vi "Measure_Power_Good.vi"(8 "error in (no error)":errorcluster, 10 "Parameters":string, 11 "reference in":refnum<class "Test_Flux_Capacitor.lvclass">) -> (0 "error out":errorcluster, 2 "Result":dbl, 3 "reference out":refnum<class "Test_Flux_Capacitor.lvclass">)   [LabVIEW 2022 SP3, in "Test_Flux_Capacitor.lvlib" / "Test_Flux_Capacitor.lvclass"]
uses:
  Test_Flux_Capacitor.lvclass
  ParameterTypes/PowerGood.ctl
  ParameterTypes/DMM_DCV.vi
  <vilib>/Analysis/baseanly.llb/Mean (DBL).vi
  <vilib>/Utility/error.llb/Trim Whitespace One-Sided.vi
  Components/SwitchBase.lvlibp/SwitchBase.lvclass
  Components/PSU_Base.lvlibp/PSU_Base.lvclass
  Components/DMM_Keysight_34980A.lvlibp/DMM_Keysight_34980A.lvclass
  <vilib>/Analysis/NI_AALBase.lvlib
  <vilib>/JDP Science/JSONtext/JSONtext.lvlib
panel:
  in  "Parameter_Type":T1={"Pre_Switch"="", "Post_Switch"="", "Wait (msec)"=0, "V"=0.0, "Chan"=0, "Enable"=FALSE, "Scale"=0.0, "DMM_DCV"={"Range "=enum."Auto", "Resolution"=enum."Default", "Samples"=1, "dt (s)"=0.0, "Timeout (s)"=10000.0}}
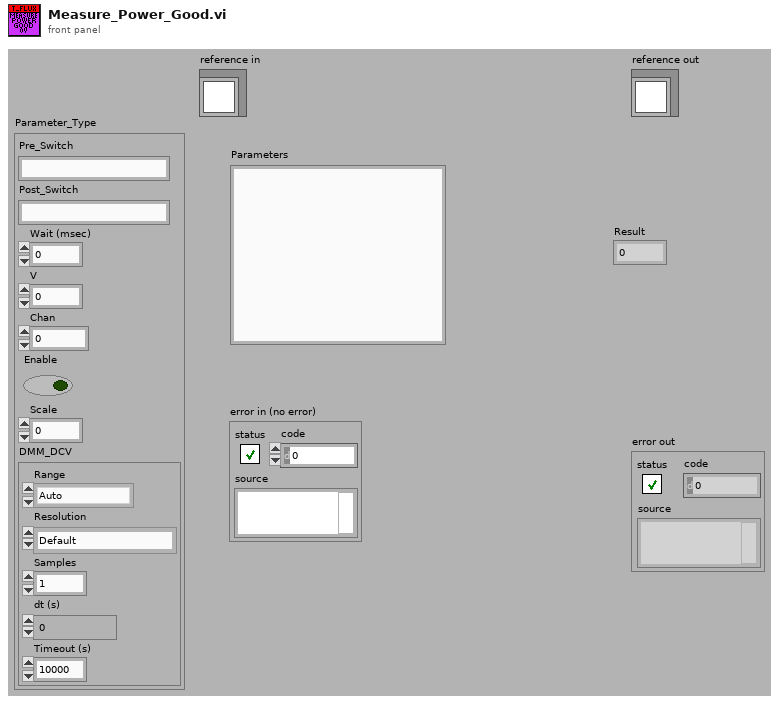
[diagram p1: front panel]
types:
  T1 = typedef "Test_Flux_Capacitor.lvlib/Test_Flux_Capacitor.lvclass/PowerGood.ctl" = cluster{"Pre_Switch":string, "Post_Switch":string, "Wait (msec)":u32, "V":dbl, "Chan":i32, "Enable":bool, "Scale":dbl, "DMM_DCV":T2}
  T2 = typedef "Test_Flux_Capacitor.lvlib/Test_Flux_Capacitor.lvclass/DMM_DCV.vi" = cluster{"Range ":enum16{"100 mV", "1 V", "10 V", "100 V", "300 V", "Auto", "Minimum", "Maximum"}, "Resolution":enum16{"4 1/2", "5 1/2", "6 1/2", "Least", "Highest", "Default"}, "Samples":u32, "dt (s)":dbl, "Timeout (s)":dbl}
  T3 = typedef "Test_Flux_Capacitor.lvlib/Test_Flux_Capacitor.lvclass/ObjectAttributes.ctl" = cluster{"Config":T4, "DMM":refnum<class "DMM_Keysight_34980A.lvclass">, "LCR":refnum<class "LCR_BK891.lvclass">, "PSU":refnum<class "PSU_Base.lvclass">, "Switch_Manager":refnum<class "SwitchBase.lvclass">, "FRAM":string, "Flux_Capacitor":refnum<class "Flux_Capacitor.lvclass">, "Frequency_Counter":refnum<class "Frequency_Counter_Base.lvclass">, "JTAG":refnum<class "JTAG_Base.lvclass">}
  T4 = typedef "Test_Flux_Capacitor.lvlib/Test_Flux_Capacitor.lvclass/Config.ctl" = cluster{"default":string}
  T5 = enum16{"100 mV", "1 V", "10 V", "100 V", "300 V", "Auto", "Minimum", "Maximum"}
  T6 = enum16{"4 1/2", "5 1/2", "6 1/2", "Least", "Highest", "Default"}
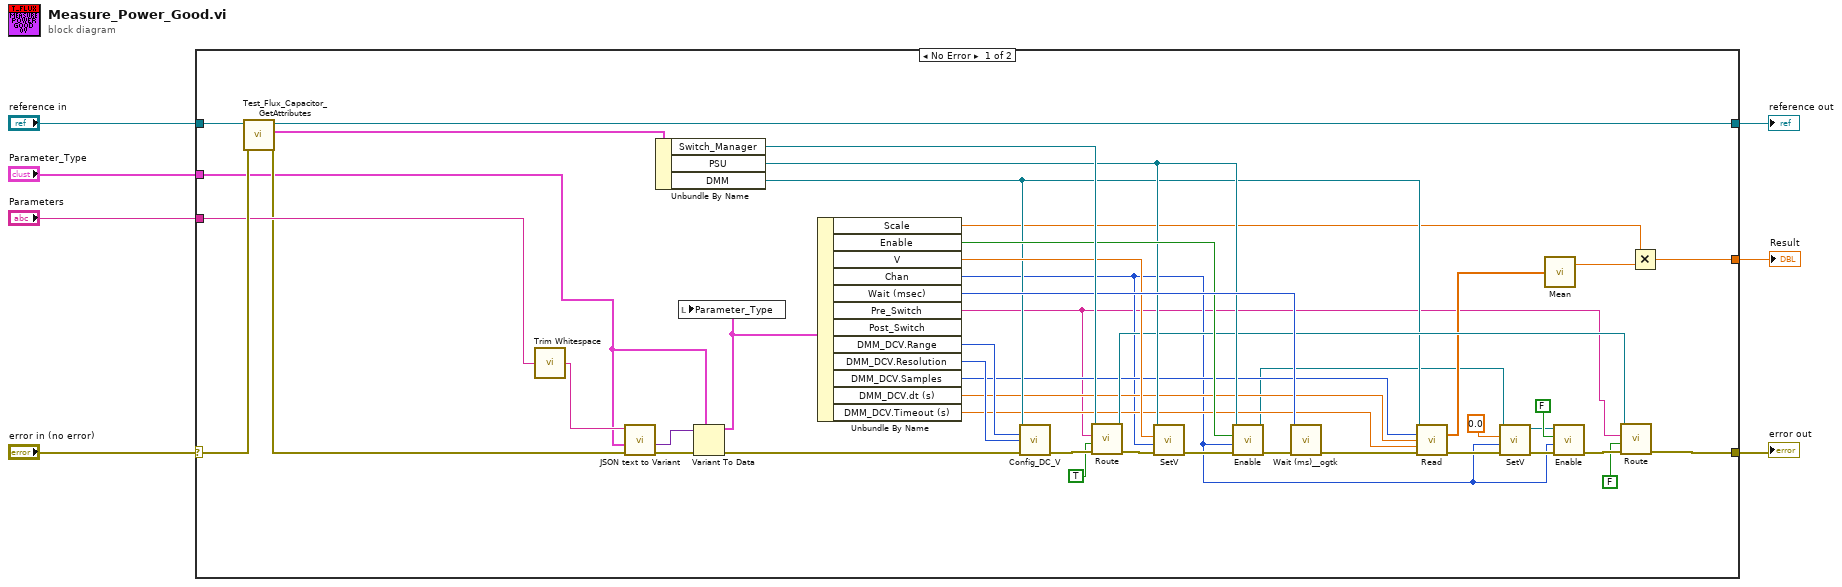
[diagram p0: block diagram]
diagram:
  n1 = case shown="No Error" "error in (no error)" {
    selector: "error in (no error)" -> [w52 w54]
    tunnel: [w36 w54] -> w6
    tunnel: [w50 w53] -> w4
    tunnel: "reference in" -> [w51 w53]
    tunnel: "Parameters" -> [w47 _]
    tunnel: "Parameter_Type" -> [w12 _]
    tunnel: [w37 _] -> w1
    frame No Error {
      n2 = call "Test_Flux_Capacitor_GetAttributes.vi"("error in (no error)"=w52, "reference in"=w51) -> ("error out"=w15:errorcluster, "Data"=w49:T3, "reference out"=w50:refnum<class "Test_Flux_Capacitor.lvclass">)  [unwired: 6 in, 1 out]
      n3 = call <vilib>:"Trim Whitespace.vi"("string"=w47) -> ("trimmed string"=w13:string)  [unwired: 1 in]
      n4 = call <vilib>:"JSON text to Variant.vi"("error in (no error)"=w15, "Data Type"=w12, "JSON"=w13) -> ("error out"=w14:errorcluster, "Variant out"=w11:variant)  [unwired: 7 in]
      n5 = Unbundle By Name(w49) -> ("Switch_Manager"=w48:refnum<class "SwitchBase.lvclass">, "PSU"=w39:refnum<class "PSU_Base.lvclass">, "DMM"=w32:refnum<class "DMM_Keysight_34980A.lvclass">)
      n6 = Variant To Data(error in=w14, type=w12, Variant=w11) -> (data=w46:T1, error out=w34:errorcluster)
      n7 = local write "Parameter_Type"(w46) -> ()
      n8 = Unbundle By Name(w46) -> ("Scale"=w26:dbl, "Enable"=w41:bool, "V"=w40:dbl, "Chan"=w17:i32, "Wait (msec)"=w45:u32, "Pre_Switch"=w10:string, "DMM_DCV.Range"=w31:T5, "DMM_DCV.Resolution"=w30:T6, "DMM_DCV.Samples"=w29:u32, "DMM_DCV.dt (s)"=w28:dbl, "DMM_DCV.Timeout (s)"=w27:dbl)  [unwired: 1 out]
      n9 = call-dynamic "Config_DC_V.vi"("reference in"=w32, "Range (5:Auto)"=w31, "Resolution (5:Default)"=w30, "error in (no error)"=w34) -> ("error out"=w33:errorcluster)  [unwired: 10 in, 1 out]
      n10 = call-dynamic "Route.vi"("error in (no error)"=w33, "Connect"=TRUE, "channel 1"=w10, "reference in"=w48) -> ("error out"=w44:errorcluster, "reference in"=w35:refnum<class "SwitchBase.lvclass">)  [unwired: 6 in]
      n11 = call-dynamic "SetV.vi"("error in (no error)"=w44, "Chan"=w17, "V"=w40, "reference in"=w39) -> ("error out"=w43:errorcluster)  [unwired: 6 in, 1 out]
      n12 = call-dynamic "Enable.vi"("error in (no error)"=w43, "Chan"=w17, "Enable"=w41, "reference in"=w39) -> ("error out"=w42:errorcluster, "reference in"=w19:refnum<class "PSU_Base.lvclass">)  [unwired: 6 in]
      n13 = call <userlib>:"Wait (ms)__ogtk.vi"("error in (no error)"=w42, "milliseconds to wait"=w45) -> ("error out"=w38:errorcluster)  [unwired: 8 in, 1 out]
      n14 = call-dynamic "Read.vi"("reference in"=w32, "Samples"=w29, "dt"=w28, "Timeout (10 s)"=w27, "error in (no error)"=w38) -> ("Measurement"=w25:dbl[], "error out"=w21:errorcluster)  [unwired: 7 in, 2 out]
      n15 = call-dynamic "SetV.vi"("error in (no error)"=w21, "Chan"=w17, "V"=0.0, "reference in"=w19) -> ("error out"=w20:errorcluster, "reference in"=w18:refnum<class "PSU_Base.lvclass">)  [unwired: 6 in]
      n16 = call-poly <vilib>:"Mean.vi"("X"=w25) -> ("mean"=w24:dbl)  [unwired: 1 out]
      n17 = call-dynamic "Enable.vi"("error in (no error)"=w20, "Chan"=w17, "Enable"=FALSE, "reference in"=w18) -> ("error out"=w23:errorcluster)  [unwired: 6 in, 1 out]
      n18 = call-dynamic "Route.vi"("error in (no error)"=w23, "Connect"=FALSE, "channel 1"=w10, "reference in"=w35) -> ("error out"=w36:errorcluster)  [unwired: 6 in, 1 out]
      n19 = Multiply(x=w26, y=w24) -> (x*y=w37:dbl)
    }
    frame Error {
    }
  }
  "Result" <- w1
  "error out" <- w6
  "reference out" <- w4
